vi "WaveFormDataGenerator.vi"(8 "error in":errorcluster, 9 "sampling info":cluster{"Fs":dbl, "#s":dbl}={"Fs"=1000.0, "#s"=100.0}, 10 "Signal Types/Classes":T1(array[ring])=[enum."Sine Wave", enum."Square Wave", enum."Triangle Wave"], 11 "Number of Waveforms per Signal Type":i32=2500) -> (0 "error out":errorcluster, 2 "Frequency":sgl[][](array[numeric]), 3 "Generated Waveform":sgl[][](array[numeric]))   [LabVIEW 2020]
uses:
  <vilib>/numeric/Random Number (Range) DBL.vi
  <vilib>/measure/NI_MABase.lvlib
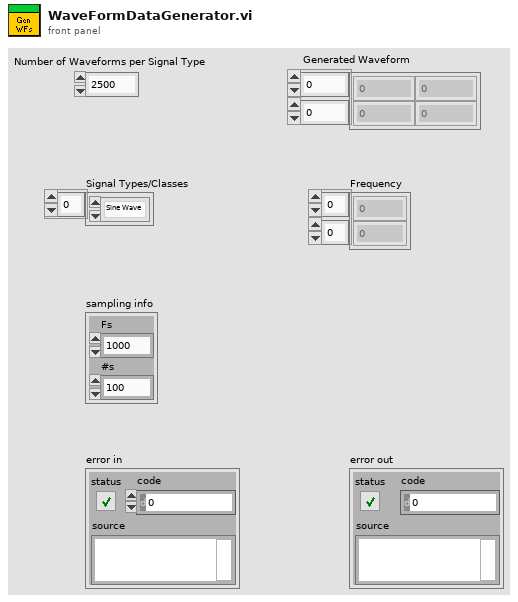
[diagram p1: front panel]
types:
  T1 = enum16{"Sine Wave", "Triangle Wave", "Square Wave", "Sawtooth Wave", "Noise"}[]
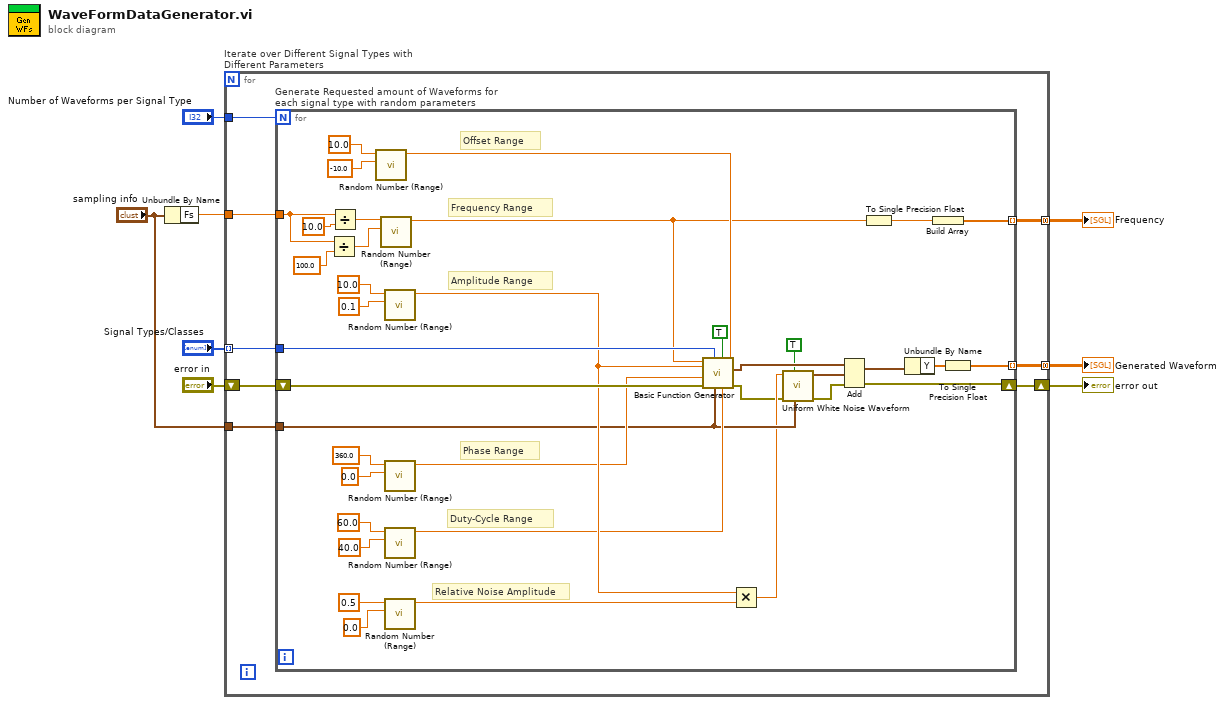
[diagram p0: block diagram]
diagram:
  n1 = Unbundle By Name("sampling info") -> ("Fs"=w8:dbl)
  n2 = for "Iterate over Different Signal Types with Different Parameters" {
    tunnel: w8 -> [w16]
    tunnel: "Number of Waveforms per Signal Type" -> [w15]
    tunnel: "sampling info" -> [w14]
    tunnel: [w11] -> w1 mode=concatenating
    tunnel: "Signal Types/Classes" -> [w10] mode=indexing
    shift-right: [w13] -> w5
    shift-left: "error in" -> [w12]
    tunnel: [w9] -> w2 mode=concatenating
    n3 = for "Generate Requested amount of Waveforms for each signal type with random parameters" {
      N: w15 -> [_]
      tunnel: [w49] -> w11 mode=indexing
      shift-right: [w52] -> w13
      shift-left: w12 -> [w53]
      tunnel: w16 -> [w46]
      tunnel: w10 -> [w48]
      tunnel: w14 -> [w31]
      tunnel: [w18] -> w9 mode=indexing
      # "Relative Noise Amplitude"
      # "Offset Range"
      # "Duty-Cycle Range"
      # "Phase Range"
      # "Amplitude Range"
      # "Frequency Range"
      n4 = Divide(x=w46, y=100.0) -> (x/y=w45:dbl)
      n5 = Divide(x=w46, y=10.0) -> (x/y=w47:dbl)
      n6 = call-poly <vilib>:"Random Number (Range).vi"("lower bound (0)"=-10.0, "upper bound (100)"=10.0) -> ("number"=w33:dbl)  [unwired: 9 in]
      n7 = call-poly <vilib>:"Random Number (Range).vi"("lower bound (0)"=w45, "upper bound (100)"=w47) -> ("number"=w20:dbl)  [unwired: 9 in]
      n8 = call-poly <vilib>:"Random Number (Range).vi"("lower bound (0)"=0.1, "upper bound (100)"=10.0) -> ("number"=w41:dbl)  [unwired: 9 in]
      n9 = call-poly <vilib>:"Random Number (Range).vi"("lower bound (0)"=0.0, "upper bound (100)"=360.0) -> ("number"=w38:dbl)  [unwired: 9 in]
      n10 = call-poly <vilib>:"Random Number (Range).vi"("lower bound (0)"=40.0, "upper bound (100)"=60.0) -> ("number"=w32:dbl)  [unwired: 9 in]
      n11 = call-poly <vilib>:"Random Number (Range).vi"("lower bound (0)"=0.0, "upper bound (100)"=0.5) -> ("number"=w27:dbl)  [unwired: 9 in]
      n12 = call <vilib>:"Basic Function Generator.vi"("offset"=w33, "square wave duty cycle (%)"=w32, "reset signal"=TRUE, "sampling info"=w31, "signal type"=w48, "error in (no error)"=w53, "phase"=w38, "amplitude"=w41, "frequency"=w20) -> ("error out"=w22:errorcluster, "signal out"=w26:waveform(dbl))  [unwired: 1 out]
      n13 = Multiply(x=w41, y=w27) -> (x*y=w24:dbl)
      n14 = call <vilib>:"Uniform White Noise Waveform.vi"("sampling info"=w31, "reset signal"=TRUE, "error in (no error)"=w22, "amplitude"=w24) -> ("error out"=w21:errorcluster, "signal out"=w23:waveform(dbl))  [unwired: 6 in]
      n15 = Add(1:w23, 2:w26, 4:w21) -> (0:w30:waveform(dbl), 3:w52:errorcluster)
      n16 = To Single Precision Float(number=w20) -> (single precision float=w19:sgl)
      n17 = Unbundle By Name(w30) -> ("Y"=w50:dbl[])
      n18 = Build Array(w19) -> (w18:sgl[])
      n19 = To Single Precision Float(number=w50) -> (single precision float=w49:sgl[])
    }
  }
  "Generated Waveform" <- w1
  "error out" <- w5
  "Frequency" <- w2
